vi "Waveform Acquisition - Create Resources (16xI16).vi"(0 "T2H FIFO":refnum<k21>, 5 "DRAM Clock":refnum<k21>, 7 "DRAM Memory":refnum<k21>, 9 "DRAM Memory Size":u32, 11 "DRAM Ready":refnum<k21>) -> (4 "Waveform Acquisition Resources":T1)   [LabVIEW 2018, in "Streaming FPGA.lvlib"]
doc: "Creates the resources for the Waveform Acquisition.\n\nThe Waveform Acquisition streams a waveform to the host through a DRAM FIFO.\n\nThis VI must be placed on the block diagram outside of any SCTLs.\n<B>T2H FIFO</B> is the Target to Host FIFO to which the waveform samples are written, this FIFO should be configured to use I16 data type and 16 elements per write operation.\n<B>DRAM Clock</B> is the clock used by the DRAM memory interface.\nThe <B>DRAM Memory</B> memory resource must use DRAM implementation and the data type must be the type provided by the <B>Data Type (B256).ctl</B> (array of 256 booleans).\nThe <B>DRAM Memory Size</B> must be the requested number of elements parameter of the <B>DRAM Memory</B> memory resource.\n<B>DRAM Ready</B> must be an FPGA Register using the boolean data type, and this register must be set to true when the DRAM is ready.\n\nThe Waveform Acquisition requires the <B>Waveform Acquisition - Process.vi</B> to be placed on the block diagram outside of any SCTLs, and to be connected to the <B>Waveform Acquisition Resources</B> output of this VI.\n\nUse the <B>Waveform Acquisition - Write.vi</B> to control the Waveform Acquisition and to write the waveform samples. This VI should be placed in an SCTL (it is not necessary to clock the SCTL by the <B>DRAM Clock</B>), and needs to be connected to the <B>Waveform Acquisition Resources</B> output of this VI."
uses:
  Streaming FPGA.lvlib
  Waveform Acquisition Resources (16xI16).ctl
  Target-Scoped FIFO (16xI16) Resource.ctl
  <vilib>/rvi/DataTransferAndStorage/Container/Common/niFpgaContainerGetUniqueNameForEmu.vi
  <vilib>/rvi/DataTransferAndStorage/Container/Common/niFpgaContainerSetEmuInfo.vi
  <vilib>/rvi/eio/common/nirviEmuReportErrorAndStop.vi
  <vilib>/rvi/LocalResourceManager/LocalResourceManager.xnode
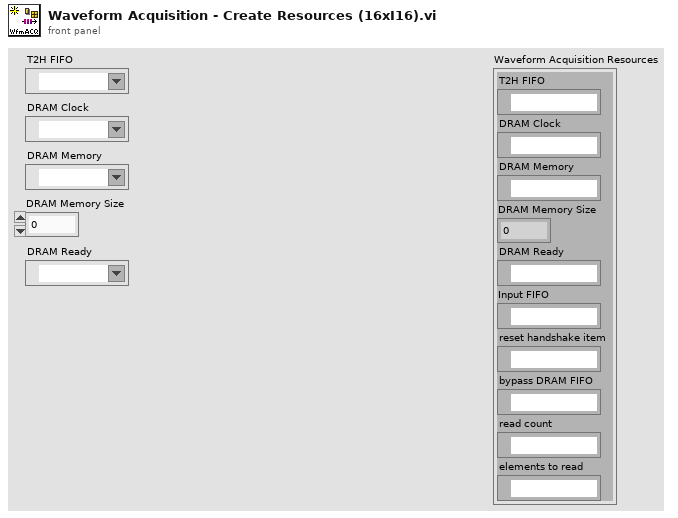
[diagram p1: front panel]
types:
  T1 = typedef "Streaming FPGA.lvlib/Waveform Acquisition Resources (16xI16).ctl" = cluster{"T2H FIFO":refnum<k21>, "DRAM Clock":refnum<k21>, "DRAM Memory":refnum<k21>, "DRAM Memory Size":u32, "DRAM Ready":refnum<k21>, "Input FIFO":T2, "reset handshake item":refnum<k21>, "bypass DRAM FIFO":refnum<k21>, "read count":refnum<k21>, "elements to read":refnum<k21>}
  T2 = typedef "Streaming FPGA.lvlib/Target-Scoped FIFO (16xI16) Resource.ctl" = refnum<k21>
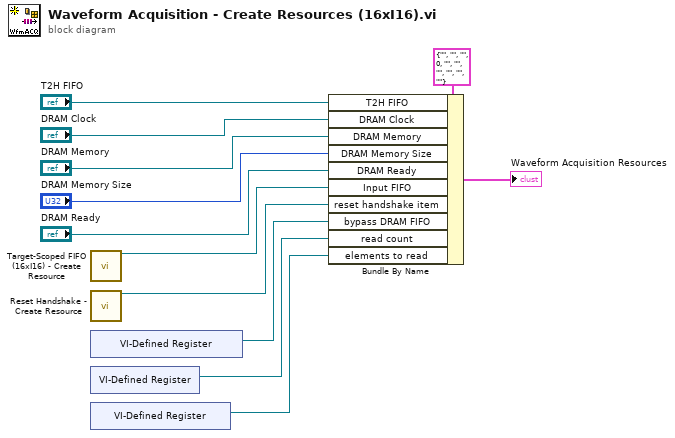
[diagram p0: block diagram]
diagram:
  n1 = call "Target-Scoped FIFO (16xI16) - Create Resource.vi"() -> ("Target-Scoped FIFO (16xI16)"=w5:T2)  [unwired: 15 in]
  n2 = call "Reset Handshake - Create Resource.vi"() -> ("reset handshake item"=w4:refnum<k21>)  [unwired: 15 in]
  n3 = xnode "VI-Defined Register"() -> ("Register Out"=w3:refnum<k21>)
  n4 = xnode "VI-Defined Register"() -> ("Register Out"=w2:refnum<k21>)
  n5 = xnode "VI-Defined Register"() -> ("Register Out"=w1:refnum<k21>)
  n6 = Bundle By Name(cluster=T1 {"T2H FIFO"="", "DRAM Clock"="", "DRAM Memory"="", "DRAM Memory Size"=0, "DRAM Ready"="", "Input FIFO"="", "reset handshake item"="", "bypass DRAM FIFO"="", "read count"="", "elements to read"=""} ("Waveform Acquisition Resources"), "T2H FIFO"="T2H FIFO", "DRAM Clock"="DRAM Clock", "DRAM Memory"="DRAM Memory", "DRAM Memory Size"="DRAM Memory Size", "DRAM Ready"="DRAM Ready", "Input FIFO"=w5, "reset handshake item"=w4, "bypass DRAM FIFO"=w3, "read count"=w2, "elements to read"=w1) -> (→"Waveform Acquisition Resources":T1)
